vi "DSF.Engine.Builder.Main Thread.vi"(8 "error in (no error)":errorcluster, 10 "Thread Parameters":refnum<class "Thread Parameters.lvclass">, 11 "Builder in":refnum<class "DSF.Engine.Builder.lvclass">) -> (0 "error out":errorcluster, 3 "Builder out":refnum<class "DSF.Engine.Builder.lvclass">)   [LabVIEW 2016, in "DSF.Engine.lvlib" / "DSF.Engine.Builder.lvclass"]
uses:
  DSF.Engine.Builder.lvclass
  Thread Parameters/Thread Parameters.lvclass
  Thread Parameters/Thread Parameters.lvclass/Thread Parameters.ctl
  <vilib>/Platform/TimedLoop/XDataNode/timing_clust.ctl
  <vilib>/Platform/TimedLoop/XDataNode/nitl_modes.ctl
  <vilib>/Platform/TimedLoop/XDataNode/wakeup.ctl
  Interface/DSF.Engine.Interface.Builder.Response Data.ctl
  Interface/DSF.Engine.Interface.Builder.Response.ctl
  Typedefs/DSF.Engine.Typedefs.Type Buffers.ctl
  <vilib>/platform/TimedLoop/XDataNode/XDataNode.xnode
  <vilib>/Platform/TimedLoop/XDataNode/XDNodeRunTimeDep.lvlib
  Interface/DSF.Engine.Interface.Builder.lvclass
  DSF.Engine.lvlib
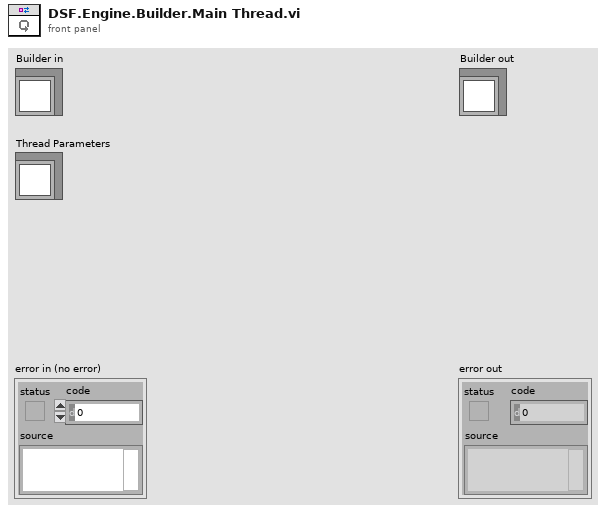
[diagram p1: front panel]
types:
  T1 = typedef "XDNodeRunTimeDep.lvlib/timing_clust.ctl" = cluster{"Expected End [f-1]":u64, "Actual End [f-1]":u64, "Finished Late? [f-1]":bool, "Expected End [i-1]":u64, "Actual End [i-1]":u64, "Finished Late? [i-1]":bool, "Expected Start [i]":u64, "Actual Start [i]":u64, "Expected Start [f]":u64, "Actual Start [f]":u64, "Source Name":string, "Structure Name":string, "Period":i64, "Deadline":i64, "Offset":i64, "Start":i64, "Priority":i32, "Timeout":i32, "Mode":T2, "Wakeup Reason":T3, "Error":errorcluster, "Source Type":string, "Secondary Source Type":string, "Global End Time":u64, "Global Start Time":u64, "Frame Duration":u64, "Iteration Duration":u64, "Assigned CPU":i32, "I/O Scan Engine Mode":u32}
  T2 = typedef "XDNodeRunTimeDep.lvlib/nitl_modes.ctl" = enum32{"No Change", "Process missed periods, maintain original phase", "Discard missed periods, maintain original phase", "Process missed periods, ignore original phase", "Discard missed periods, ignore original phase"}
  T3 = typedef "XDNodeRunTimeDep.lvlib/wakeup.ctl" = enum32{"Normal", "Aborted", "Asynchronous wakeup", "Timing source error", "Timed loop error", "Timeout"}
  T4 = typedef "DSF.Engine.lvlib/DSF.Engine.Typedefs.Type Buffers.ctl" = cluster{"Bool":bool[], "SGL":sgl[], "DBL":dbl[], "I8":i8[], "I16":i16[], "I32":i32[], "I64":i64[], "U8":u8[], "U16":u16[], "U32":u32[], "U64":u64[]}
  T5 = typedef "DSF.Engine.lvlib/DSF.Engine.Interface.Builder.lvclass/DSF.Engine.Interface.Builder.Response Data.ctl" = cluster{"Response":T6, "arg1":i32, "arg2":i32, "arg3":i32, "arg4":i32}
  T6 = typedef "DSF.Engine.lvlib/DSF.Engine.Interface.Builder.lvclass/DSF.Engine.Interface.Builder.Response.ctl" = enum8{"General Ack", "Initialize Complete", "Build Complete", "Parse Complete", "Shutdown Ack"}
  T7 = typedef "DSF.Engine.lvlib/DSF.Engine.Interface.Builder.lvclass/DSF.Engine.Interface.Builder.Command.ctl" = enum8{"Idle", "Initialize", "Build Buffer", "Parse Buffer", "Shutdown"}
  T8 = typedef "DSF.Engine.lvlib/DSF.Engine.Interface.Builder.lvclass/DSF.Engine.Interface.Builder.Command Data.ctl" = cluster{"Command":T7, "arg1":i32, "arg2":i32, "arg3":i32, "arg4":i32}
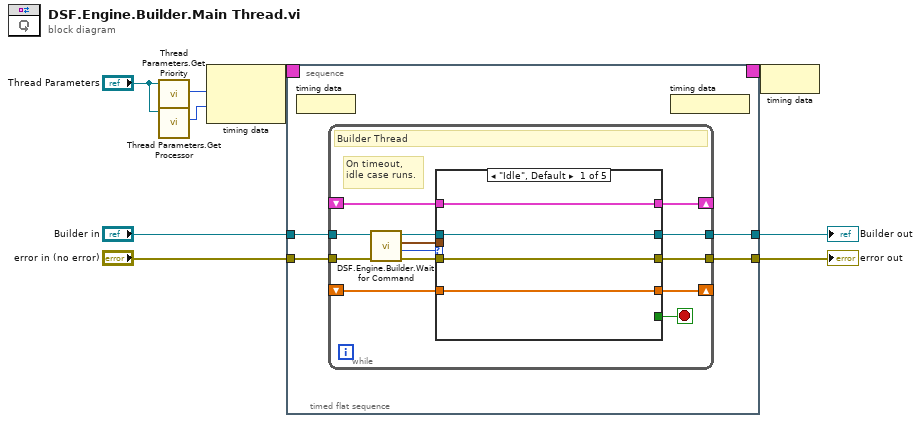
[diagram p0: block diagram]
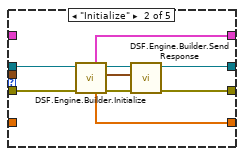
[diagram p2: hidden frame]
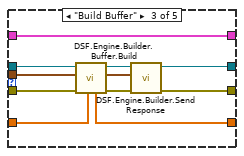
[diagram p3: hidden frame]
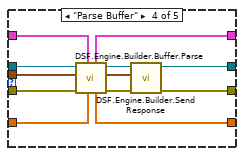
[diagram p4: hidden frame]
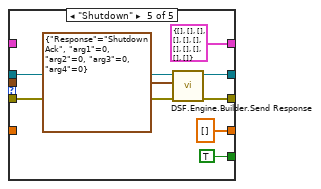
[diagram p5: hidden frame]
diagram:
  n1 = call "Thread Parameters.Get Priority.vi"("Thread Parameters in"="Thread Parameters") -> ("Priority"=w6:i32)  [unwired: 9 in, 1 out]
  n2 = call "Thread Parameters.Get Processor.vi"("Thread Parameters in"="Thread Parameters") -> ("Processor"=w5:i32)  [unwired: 9 in, 1 out]
  n3 = node-c288(w6, w5) -> (w8:T1)
  n4 = timed-sequence {
    timing: w8 -> [_]
    timing-out: [_] -> w7
    tunnel: "Builder in" -> [w12]
    tunnel: [w13] -> w4
    tunnel: "error in (no error)" -> [w11]
    tunnel: [w10] -> w2
    n5 = timed-flat-sequence {
      tunnel: [w17] -> w13
      tunnel: w12 -> [w15]
      tunnel: w11 -> [w16]
      tunnel: [w14] -> w10
      n6 = node-c288() -> ()  [unwired: 1 in]
      n7 = while {
        tunnel: w15 -> [w27]
        tunnel: [w30] -> w17
        tunnel: w16 -> [w32]
        tunnel: [w28] -> w14
        shift-right: [w25] -> _
        shift-left: _ -> [w20]
        shift-right: [w24] -> _
        shift-left: _ -> [w23]
        stop <- w26 stop-if-true
        # "On timeout, idle case runs."
        # "Builder Thread"
        n8 = call "DSF.Engine.Builder.Wait for Command.vi"("error in (no error)"=w32, "Builder in"=w27) -> ("error out"=w29:errorcluster, "command action"=w21:T7, "command data"=w22:T8, "Builder out"=w31:refnum<class "DSF.Engine.Builder.lvclass">)  [unwired: 6 in]
        n9 = case shown="\"Idle\", Default" w21 {
          tunnel: w31 -> [w36 w45 w53 w64 w76]
          tunnel: [w36 w41 w48 w59 w75] -> w30
          tunnel: w29 -> [w35 w44 w51 w63 w72]
          tunnel: [w35 w40 w47 w58 w74] -> w28
          tunnel: [_ _ _ _ TRUE] -> w26
          tunnel: w20 -> [w34 _ w54 w68 _]
          tunnel: [w34 w43 w54 w67 T4 {"Bool"=[], "SGL"=[], "DBL"=[], "I8"=[], "I16"=[], "I32"=[], "I64"=[], "U8"=[], "U16"=[], "U32"=[], "U64"=[]} ("Data Type Buffers")] -> w25
          tunnel: w22 -> [_ _ w52 w62 _]
          tunnel: [w33 w42 w55 w65 dbl[] [] ("VS Channel Buffer out")] -> w24
          tunnel: w23 -> [w33 _ w56 w66 _]
          frame "Idle", Default {
          }
          frame "Initialize" {
            n10 = call "DSF.Engine.Builder.Initialize.vi"("error in (no error)"=w44, "Builder in"=w45) -> ("error out"=w38:errorcluster, "response"=w37:T5, "Builder out"=w39:refnum<class "DSF.Engine.Builder.lvclass">, "VS Channels Buffer"=w42:dbl[], "Data Type Buffers"=w43:T4)  [unwired: 5 in]
            n11 = call "DSF.Engine.Builder.Send Response.vi"("error in (no error)"=w38, "response"=w37, "Builder in"=w39) -> ("error out"=w40:errorcluster, "Builder out"=w41:refnum<class "DSF.Engine.Builder.lvclass">)  [unwired: 7 in]
          }
          frame "Build Buffer" {
            n12 = call "DSF.Engine.Builder.Buffer.Build.vi"("VS Channel Buffer in"=w56, "error in (no error)"=w51, "command"=w52, "Builder in"=w53) -> ("error out"=w50:errorcluster, "response"=w46:T5, "Builder out"=w49:refnum<class "DSF.Engine.Builder.lvclass">, "VS Channel Buffer out"=w55:dbl[])  [unwired: 4 in]
            n13 = call "DSF.Engine.Builder.Send Response.vi"("error in (no error)"=w50, "response"=w46, "Builder in"=w49) -> ("error out"=w47:errorcluster, "Builder out"=w48:refnum<class "DSF.Engine.Builder.lvclass">)  [unwired: 7 in]
          }
          frame "Parse Buffer" {
            n14 = call "DSF.Engine.Builder.Buffer.Parse.vi"("VS Channel Buffer in"=w66, "Data Type Buffers in"=w68, "error in (no error)"=w63, "command"=w62, "Builder in"=w64) -> ("error out"=w60:errorcluster, "response"=w57:T5, "Builder out"=w61:refnum<class "DSF.Engine.Builder.lvclass">, "VS Channel Buffer out"=w65:dbl[], "Data Type Buffers out"=w67:T4)  [unwired: 2 in]
            n15 = call "DSF.Engine.Builder.Send Response.vi"("error in (no error)"=w60, "response"=w57, "Builder in"=w61) -> ("error out"=w58:errorcluster, "Builder out"=w59:refnum<class "DSF.Engine.Builder.lvclass">)  [unwired: 7 in]
          }
          frame "Shutdown" {
            n16 = call "DSF.Engine.Builder.Send Response.vi"("error in (no error)"=w72, "response"=T5 {"Response"=enum."Shutdown Ack", "arg1"=0, "arg2"=0, "arg3"=0, "arg4"=0}, "Builder in"=w76) -> ("error out"=w74:errorcluster, "Builder out"=w75:refnum<class "DSF.Engine.Builder.lvclass">)  [unwired: 7 in]
          }
        }
      }
      n17 = node-c288() -> ()  [unwired: 1 out]
    }
  }
  "error out" <- w2
  "Builder out" <- w4
  n18 = node-c288(w7) -> ()
